vi "Scrub.vi"(8 "error in":errorcluster, 10 "Input String":string, 11 "Scrubber in":refnum<class "Scrubber.lvclass">) -> (0 "error out":errorcluster, 2 "Scrubbed String":string, 3 "Scrubber out":refnum<class "Scrubber.lvclass">)   [LabVIEW 2020, in "Approval Tests.lvlib" / "Scrubber.lvclass"]
uses:
  Scrubber.lvclass
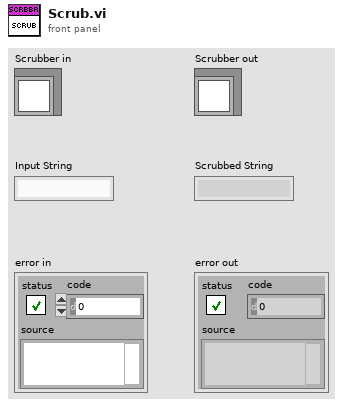
[diagram p1: front panel]
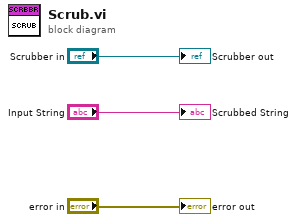
[diagram p0: block diagram]
diagram:
  "error out" <- "error in"
  "Scrubber out" <- "Scrubber in"
  "Scrubbed String" <- "Input String"
